vi "Average.vi"(10 "Array":dbl[](array[numeric])) -> (1 "Standard Deviation":dbl, 2 "Average":dbl)   [LabVIEW 2014]
panel:
  out "Numeric":dbl
  out "newArray":dbl[](array[numeric])
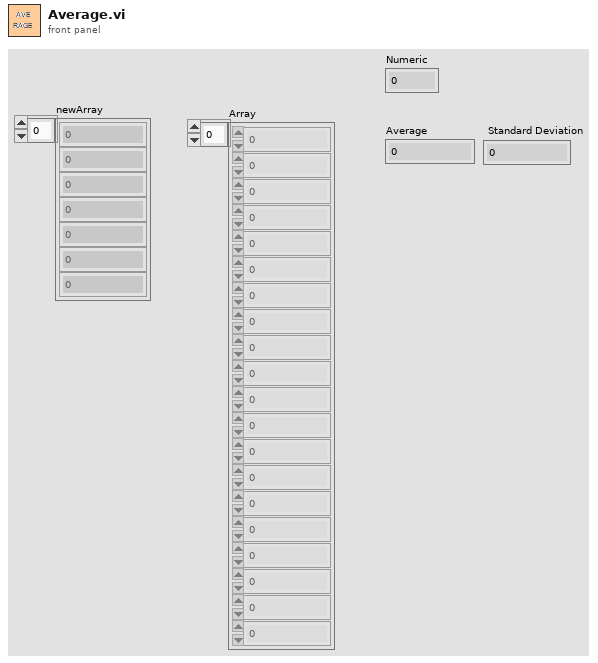
[diagram p1: front panel]
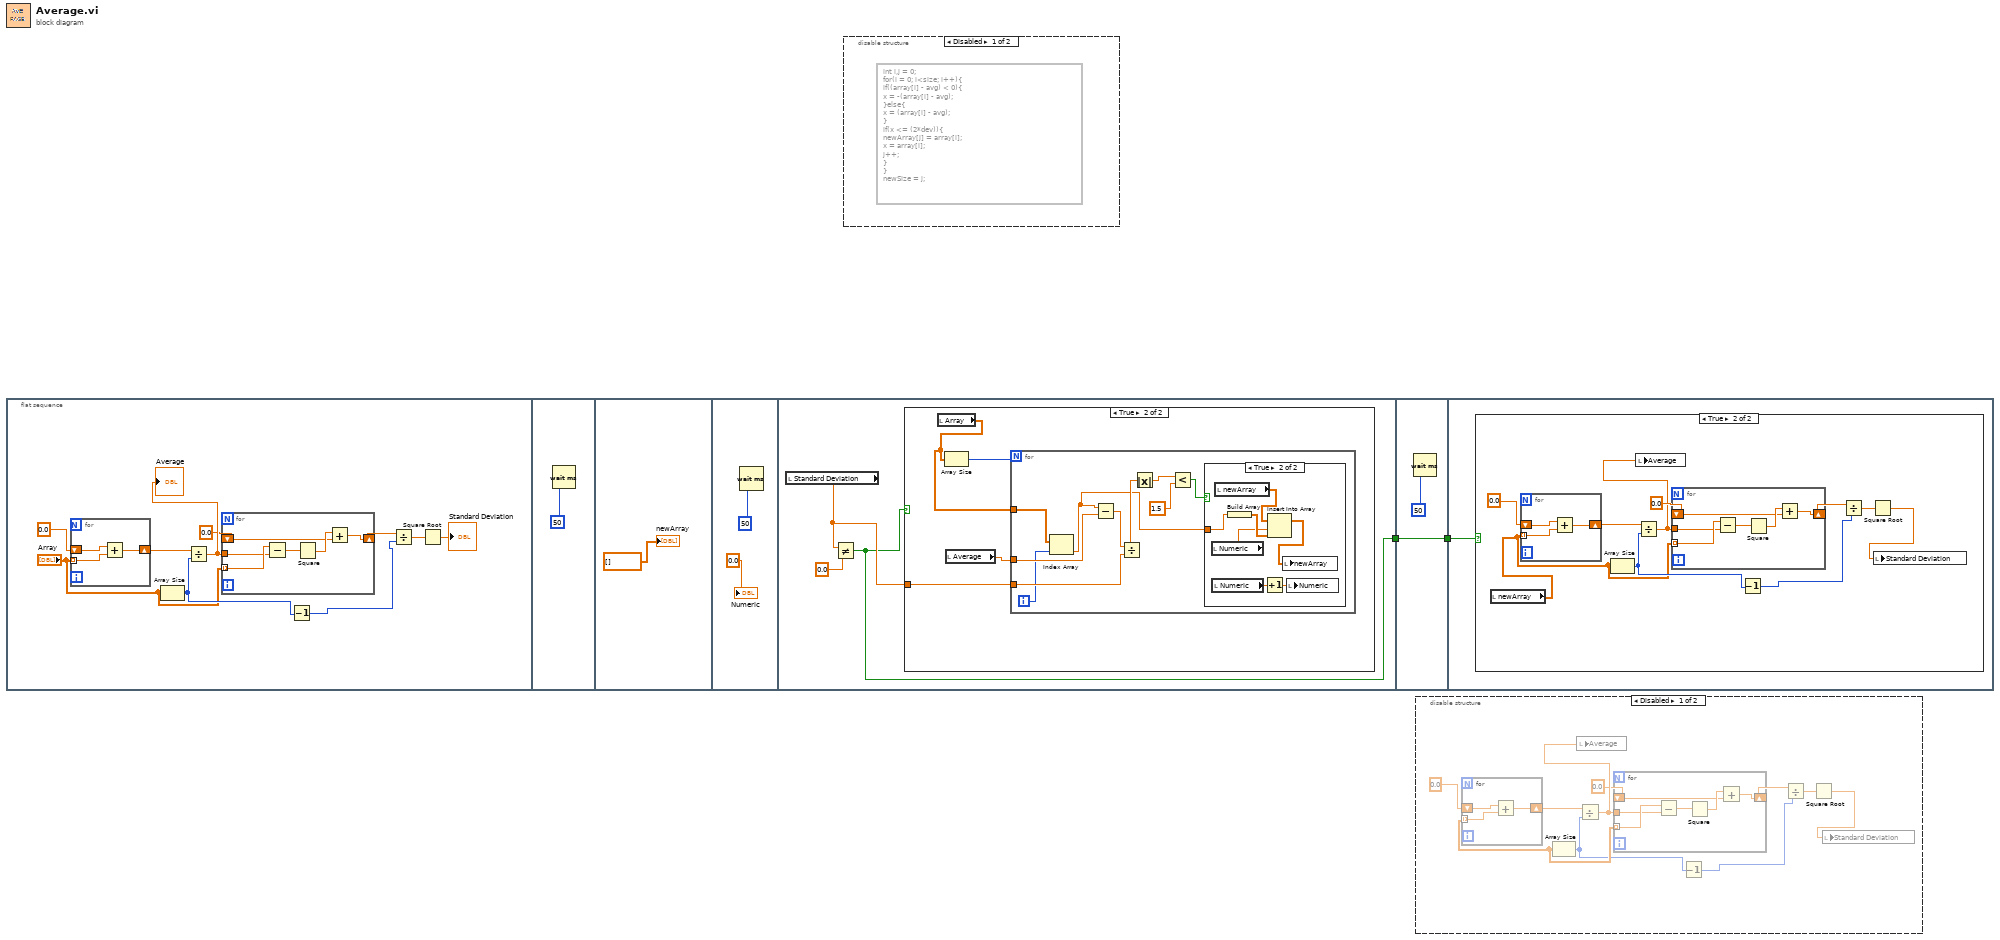
[diagram p0: block diagram]
diagram:
  n1 = flat-sequence {
    tunnel: [w26] -> w2
    tunnel: w2 -> [w51]
    tunnel: [w51] -> w1
    tunnel: w1 -> [w52]
    frame #0 {
      n2 = for {
        tunnel: "Array" -> [w21] mode=indexing
        shift-right: [w20] -> w3
        shift-left: 0.0 -> [w19]
        n3 = Add(x=w19, y=w21) -> (x+y=w20:dbl)
      }
      n4 = Array Size(array="Array") -> (size(s)=w8:i32)
      n5 = Divide(x=w3, y=w8) -> (x/y=w11:dbl)
      "Average" <- w11
      n6 = for {
        shift-right: [w18] -> w9
        shift-left: 0.0 -> [w13]
        tunnel: "Array" -> [w17] mode=indexing
        tunnel: w11 -> [w16]
        n7 = Subtract(x=w17, y=w16) -> (x-y=w15:dbl)
        n8 = Square(x=w15) -> (x^2=w14:dbl)
        n9 = Add(x=w14, y=w13) -> (x+y=w18:dbl)
      }
      n10 = Decrement(x=w8) -> (x-1=w12:i32)
      n11 = Divide(x=w9, y=w12) -> (x/y=w6:dbl)
      n12 = Square Root(x=w6) -> (sqrt(x)=→"Standard Deviation":dbl)
    }
    frame #1 {
      n13 = Wait (ms)(milliseconds to wait=u32 50) -> ()  [unwired: 1 out]
    }
    frame #2 {
      "newArray" <- dbl[] []
    }
    frame #3 {
      n14 = Wait (ms)(milliseconds to wait=u32 50) -> ()  [unwired: 1 out]
      "Numeric" <- 0.0 ("Numeric")
    }
    frame #4 {
      n15 = local read "Standard Deviation"() -> (w27:dbl)
      n16 = Not Equal?(x=w27, y=0.0) -> (x != y?=w26:bool)
      n17 = case shown="True" w26 {
        tunnel: w27 -> [_ w30]
        frame False {
        }
        frame True {
          n18 = local read "Array"() -> (w31:dbl[])
          n19 = Array Size(array=w31) -> (size(s)=w29:i32)
          n20 = local read "Average"() -> (w32:dbl)
          n21 = for {
            N: w29 -> [_]
            tunnel: w31 -> [w42]
            tunnel: w32 -> [w41]
            tunnel: w30 -> [w35]
            i -> [w33]
            n22 = Index Array(array=w42, index=w33) -> (element=w34:dbl)
            n23 = Subtract(x=w34, y=w41) -> (x-y=w40:dbl)
            n24 = Divide(x=w40, y=w35) -> (x/y=w39:dbl)
            n25 = Absolute Value(x=w39) -> (abs(x)=w36:dbl)
            n26 = Less?(x=w36, y=1.5) -> (x < y?=w37:bool)
            n27 = case shown="True" w37 {
              tunnel: w34 -> [_ w49]
              frame False {
              }
              frame True {
                n28 = local read "Numeric"() -> (w45:dbl)
                n29 = local read "Numeric"() -> (w43:dbl)
                n30 = local read "newArray"() -> (w47:dbl[])
                n31 = Build Array(w49) -> (w46:dbl[])
                n32 = Increment(x=w43) -> (x+1=w44:dbl)
                n33 = Insert Into Array(array=w47, index=w45, new element=w46) -> (w48:dbl[])
                n34 = local write "newArray"(w48) -> ()
                n35 = local write "Numeric"(w44) -> ()
              }
            }
          }
        }
      }
    }
    frame #5 {
      n36 = Wait (ms)(milliseconds to wait=u32 50) -> ()  [unwired: 1 out]
    }
    frame #6 {
      n37 = case shown="True" w52 {
        frame False {
        }
        frame True {
          n38 = local read "newArray"() -> (w53:dbl[])
          n39 = for {
            tunnel: w53 -> [w71] mode=indexing
            shift-right: [w70] -> w56
            shift-left: 0.0 -> [w69]
            n40 = Add(x=w69, y=w71) -> (x+y=w70:dbl)
          }
          n41 = Array Size(array=w53) -> (size(s)=w59:i32)
          n42 = Divide(x=w56, y=w59) -> (x/y=w55:dbl)
          n43 = local write "Average"(w55) -> ()
          n44 = for {
            shift-right: [w68] -> w60
            shift-left: 0.0 -> [w63]
            tunnel: w53 -> [w67] mode=indexing
            tunnel: w55 -> [w66]
            n45 = Subtract(x=w67, y=w66) -> (x-y=w65:dbl)
            n46 = Square(x=w65) -> (x^2=w64:dbl)
            n47 = Add(x=w64, y=w63) -> (x+y=w68:dbl)
          }
          n48 = Decrement(x=w59) -> (x-1=w62:i32)
          n49 = Divide(x=w60, y=w62) -> (x/y=w58:dbl)
          n50 = Square Root(x=w58) -> (sqrt(x)=w54:dbl)
          n51 = local write "Standard Deviation"(w54) -> ()
        }
      }
    }
  }
  n52 = disable-structure shown="Disabled" {
    frame Disabled {
      n53 = formula code="int i,j = 0;\nfor(i = 0; i<size; i++){\nif((array[i] - avg) < 0){\nx = -(array[i] - avg);\n}else{\nx = (array[i] - avg);\n}\nif(x <= (2*dev)){\nnewArray[j] = array[i];\nx = array[i];\nj++;\n}\n}\nnewSize = j;"() -> ()
    }
    frame Enabled {
    }
  }
  n54 = disable-structure shown="Disabled" {
    frame Disabled {
      n55 = Array Size() -> (array=w81:dbl[], size(s)=w75:i32)
      n56 = for {
        tunnel: w81 -> [w90] mode=indexing
        shift-right: [w89] -> w78
        shift-left: 0.0 -> [w88]
        n57 = Add(x=w88, y=w90) -> (x+y=w89:dbl)
      }
      n58 = Divide(x=w78, y=w75) -> (x/y=w79:dbl)
      n59 = local write "Average"(w79) -> ()
      n60 = for {
        shift-right: [w87] -> w74
        shift-left: 0.0 -> [w82]
        tunnel: w81 -> [w86] mode=indexing
        tunnel: w79 -> [w85]
        n61 = Subtract(x=w86, y=w85) -> (x-y=w84:dbl)
        n62 = Square(x=w84) -> (x^2=w83:dbl)
        n63 = Add(x=w83, y=w82) -> (x+y=w87:dbl)
      }
      n64 = Decrement(x=w75) -> (x-1=w72:i32)
      n65 = Divide(x=w74, y=w72) -> (x/y=w76:dbl)
      n66 = Square Root(x=w76) -> (sqrt(x)=w80:dbl)
      n67 = local write "Standard Deviation"(w80) -> ()
    }
    frame Enabled {
    }
  }
